vi "OpenConnection.vi"(8 "error in (no error)":errorcluster, 9 "Timeout (ms)":u32=5000 min=1, 10 "Connection Params":T1={"Vid"=0, "Pid"=0, "Device Index"=0, "u32_I2Cclk"=100} {"u32_I2Cclk" min=100 max=4000 step=1 format="%d Kbps"; "Pid" format="%.0x"; "Vid" format="%.0x"}, 11 "I2COUSBSim in":refnum<class "I2COUSBSim.lvclass">) -> (0 "error out":errorcluster, 3 "I2COUSBSim out":refnum<class "I2COUSBSim.lvclass">)   [LabVIEW 2020, in "I2COUSB.lvlib" / "I2COUSBSim.lvclass"]
doc: "Open connection"
uses:
  I2COUSBSim.lvclass
  II2COUSB/II2COUSB/ConnectionParams.ctl
  I2COUSBSim.lvclass/I2COUSBSim.ctl
  II2COUSB/II2COUSB/II2COUSB.lvclass
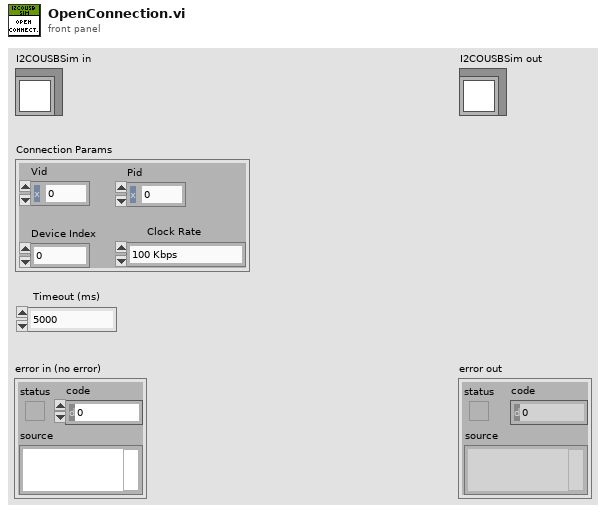
[diagram p1: front panel]
types:
  T1 = typedef "II2COUSB.lvlib/II2COUSB.lvclass/ConnectionParams.ctl" = cluster{"Vid":u16, "Pid":u16, "Device Index":u32, "u32_I2Cclk":u32}
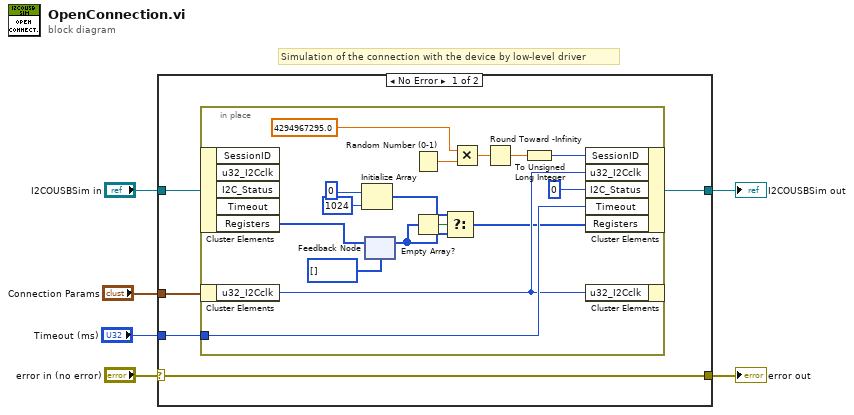
[diagram p0: block diagram]
diagram:
  # "Simulation of the connection with the device by low-level driver"
  n1 = case shown="No Error" "error in (no error)" {
    selector: "error in (no error)" -> [w11 w28]
    tunnel: "I2COUSBSim in" -> [w10 w29]
    tunnel: [w9 w29] -> w5
    tunnel: [w11 w28] -> w3
    tunnel: "Timeout (ms)" -> [w8 _]
    tunnel: "Connection Params" -> [w7 _]
    frame No Error {
      n2 = in-place {
        in-place-border: w8 -> [w27]
        n3 = in-place-cluster #1(w10) -> ("Registers"=w19:u8[])  [unwired: 4 out]
        n4 = in-place-cluster #2(w7) -> ("u32_I2Cclk"=w25:u32)
        n5 = Initialize Array(u8 0 ("Register"), 1024 ("dimension size")) -> (w14:u8[])
        n6 = feedback-in #3(w19) -> ()
        n7 = feedback #3(u8[] [] ("Registers")) -> (w12:u8[])
        n8 = Random Number (0-1)() -> (number: 0 to 1=w24:dbl)
        n9 = Empty Array?(array=w12) -> (empty?=w17:bool)
        n10 = Select(t=w14, s=w17, f=w12) -> (s? t:f=w13:u8[])
        n11 = Multiply(x=4294967295.0, y=w24) -> (x*y=w22:dbl)
        n12 = Round Toward -Infinity(1:w22) -> (0:w21:dbl)
        n13 = To Unsigned Long Integer(number=w21) -> (unsigned 32bit integer=w20:u32)
        n14 = in-place-cluster #1("SessionID"=w20, "u32_I2Cclk"=w25, "I2C_Status"=u8 0 ("eFT260_Status"), "Timeout"=w27, "Registers"=w13) -> (w9:refnum<class "I2COUSBSim.lvclass">)
        n15 = in-place-cluster #2("u32_I2Cclk"=w25) -> ()  [unwired: 1 out]
      }
    }
    frame Error {
    }
  }
  "error out" <- w3
  "I2COUSBSim out" <- w5
